vi "3.1.vi"() -> ()   [LabVIEW 2014]
panel:
  out "Warning Y/N":bool
  out "Warning Text":string
  in  "Min Temp":dbl
  in  "Max Temp":dbl
  in  "Current Temp":dbl
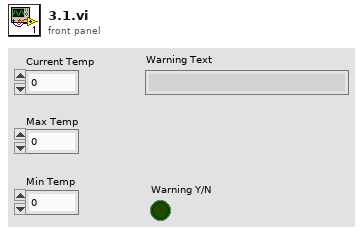
[diagram p1: front panel]
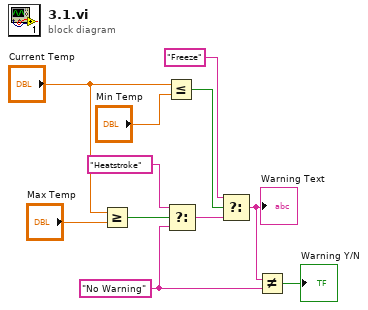
[diagram p0: block diagram]
diagram:
  w4 = "No Warning"
  n1 = Greater Or Equal?(x="Current Temp", y="Max Temp") -> (x >= y?=w3:bool)
  n2 = Less Or Equal?(x="Current Temp", y="Min Temp") -> (x <= y?=w11:bool)
  n3 = Select(t="Heatstroke", s=w3, f=w4) -> (s? t:f=w7:string)
  n4 = Select(t="Freeze", s=w11, f=w7) -> (s? t:f=w6:string)
  "Warning Text" <- w6
  n5 = Not Equal?(x=w6, y=w4) -> (x != y?=→"Warning Y/N":bool)
